vi "Configure Application Log.vi"(4 "Configuration.Level":T1=enum."Debug", 6 "Configuration.Enabled":bool=TRUE, 7 "Configuration.Call Chain":bool, 8 "error in (no error)":errorcluster, 11 "Asynchronous Application Log in":refnum<class "Asynchronous Application Log.lvclass">) -> (0 "error out":errorcluster, 3 "Asynchronous Application Log out":refnum<class "Asynchronous Application Log.lvclass">)   [LabVIEW 2016, in "Stream Log.lvlib" / "Asynchronous Application Log.lvclass"]
doc: "--\nCopyright © 2017 Composed SystemsI All rights reserved.\n\nAuthor: Jon McBee <jon.mcbee@composed.io>\n\nThis library is provided \"AS IS\" ,WITHOUT WARRANTIES OR\nCONDITIONS OF ANY KIND, either express or implied.\n\nComposed Systems -- composed.io\n\nStream 0.0.1.1\nJon McBee - Composed Systems\nCopyright (c) 2017, Composed Systems"
uses:
  <userlib>/Composed Systems/Stream/Log/Asynchronous Application Log/Asynchronous Application Log.lvclass
  <userlib>/Composed Systems/Stream/Log/Application Log/Log Level.ctl
  <userlib>/Composed Systems/Stream/Log/Application Log/Application Log.lvclass
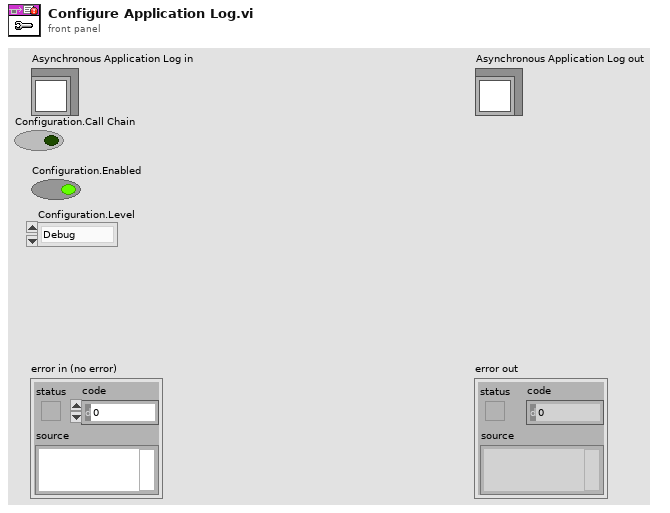
[diagram p1: front panel]
types:
  T1 = typedef "Stream Log.lvlib/Application Log.lvclass/Log Level.ctl" = enum16{"Imperative", "Major", "Minor", "Debug", "Off"}
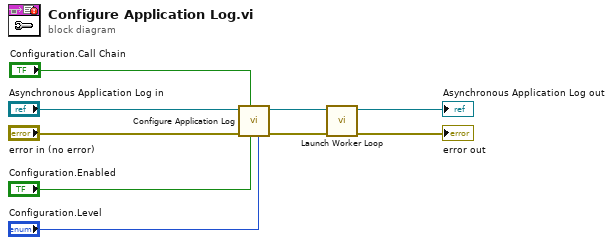
[diagram p0: block diagram]
diagram:
  n1 = call-parent "Configure Application Log.vi"("Configuration.Level"="Configuration.Level", "Configuration.Enabled"="Configuration.Enabled", "Configuration.Call Chain"="Configuration.Call Chain", "error in (no error)"="error in (no error)", "Application Log in"="Asynchronous Application Log in") -> ("error out"=w3:errorcluster, "Application Log out"=w5:refnum<class "Asynchronous Application Log.lvclass">)  [unwired: 5 in]
  n2 = call <userlib>:"Launch Worker Loop.vi"("error in (no error)"=w3, "Asynchronous Application Log in"=w5) -> ("error out"=→"error out":errorcluster, "Asynchronous Application Log out"=→"Asynchronous Application Log out":refnum<class "Asynchronous Application Log.lvclass">)  [unwired: 8 in]
